vi "QuadraticScaling.vi"(8 "error in (no error)":errorcluster, 9 "RawValCh2":dbl, 10 "RawValCh1":dbl, 11 "Gentec Slink in":refnum<class "Gentec Slink.lvclass">) -> (0 "error out":errorcluster, 1 "ScaledValueCh2":dbl, 2 "ScaledValueCh1":dbl, 3 "Gentec Slink out":refnum<class "Gentec Slink.lvclass">)   [LabVIEW 2020, in "Gentec Slink.lvclass"]
uses:
  Gentec Slink.lvclass
  Gentec Slink.lvclass/Gentec Slink.ctl
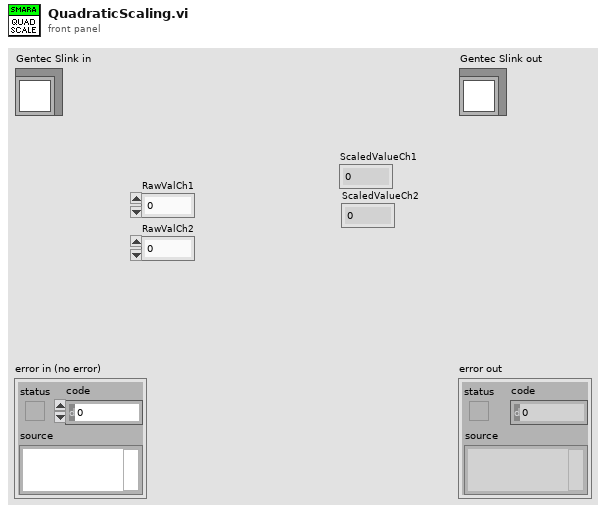
[diagram p1: front panel]
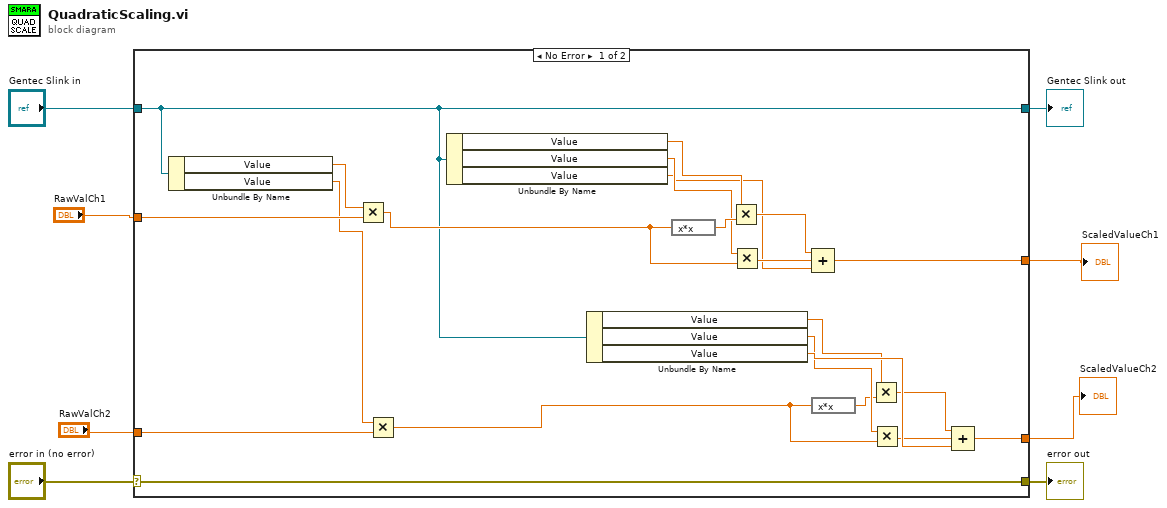
[diagram p0: block diagram]
diagram:
  n1 = case shown="No Error" "error in (no error)" {
    selector: "error in (no error)" -> [w30 w34]
    tunnel: [w30 w34] -> w7
    tunnel: [w12 w33] -> w5
    tunnel: "Gentec Slink in" -> [w12 w33]
    tunnel: "RawValCh1" -> [w28 w32]
    tunnel: "RawValCh2" -> [w26 w31]
    tunnel: [w10 w32] -> w2
    tunnel: [w9 w31] -> w1
    frame No Error {
      n2 = Unbundle By Name(w12) -> ("Value"=w29:dbl, "Value"=w27:dbl)
      n3 = Multiply(x=w29, y=w28) -> (x*y=w23:dbl)
      n4 = Multiply(x=w27, y=w26) -> (x*y=w11:dbl)
      n5 = Unbundle By Name(w12) -> ("Value"=w24:dbl, "Value"=w22:dbl, "Value"=w19:dbl)
      n6 = Unbundle By Name(w12) -> ("Value"=w14:dbl, "Value"=w15:dbl, "Value"=w18:dbl)
      n7 = expression code="x*x"(w23) -> (w25:dbl)
      n8 = Multiply(x=w24, y=w25) -> (x*y=w21:dbl)
      n9 = Multiply(x=w22, y=w23) -> (x*y=w20:dbl)
      n10 = Compound Arithmetic op=ADD(w21, w20, w19) -> (w10:dbl)
      n11 = expression code="x*x"(w11) -> (w13:dbl)
      n12 = Multiply(x=w14, y=w13) -> (x*y=w16:dbl)
      n13 = Multiply(x=w15, y=w11) -> (x*y=w17:dbl)
      n14 = Compound Arithmetic op=ADD(w16, w17, w18) -> (w9:dbl)
    }
    frame Error {
    }
  }
  "error out" <- w7
  "Gentec Slink out" <- w5
  "ScaledValueCh1" <- w2
  "ScaledValueCh2" <- w1
